vi "Fetch Multi Eval Meas ACLR Detected Allocation Results.vi"(8 "error in (no error)":errorcluster, 10 "Instance (1)":T2=1, 11 "VISA resource name":refnum<visa-resource-name>) -> (0 "error out":errorcluster, 1 "Detected Allocation":T1, 2 "Reliability":i32, 3 "VISA resource name out":refnum<visa-resource-name>)   [LabVIEW 2020, in "Rohde&Schwarz CMWXP NR FR1 Measurement.lvlib"]
doc: "Returns the ACLR detected allocation for the measured slot.\n\nIf the same slot is measured by the individual measurements, all commands yield the same result. If different statistic counts are defined for the modulation, ACLR and spectrum emission mask measurements, different slots can be measured and different results can be returned by the individual commands.\n\nAttribute:\nRSCMWXPNRFR1M_ATTR_FETCH_MULTI_EVAL_MEAS_ACLR_DETECTED_ALLOCATION_RESULTS\n\nRemote-control command:\nFETCh:NRSub:MEAS<i>:MEValuation:ACLR:DALLocation?"
uses:
  <instrlib>/Rohde&Schwarz CMWXP NR FR1 Measurement/Rohde&Schwarz CMWXP NR FR1 Measurement.lvlib
  <instrlib>/Rohde&Schwarz CMWXP NR FR1 Measurement/Private/_Instance.ctl
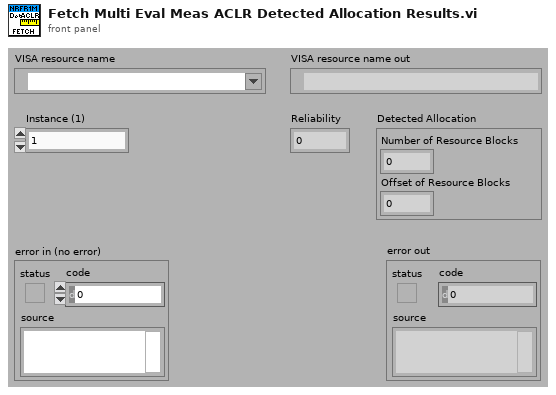
[diagram p1: front panel]
types:
  T1 = cluster{"Number of Resource Blocks":i32, "Offset of Resource Blocks":i32}
  T2 = typedef "Rohde&Schwarz CMWXP NR FR1 Measurement.lvlib/_Instance.ctl" = i32
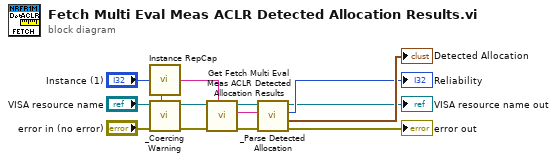
[diagram p0: block diagram]
diagram:
  n1 = call <instrlib>:"Instance RepCap.vi"("Instance In"="Instance (1)") -> ("In Range?"=w11:bool, "RepCap Identifier Out"=w9:string)  [unwired: 1 in]
  n2 = call <instrlib>:"_Coercing Warning.vi"("In Range?"=w11, "error in (no error)"="error in (no error)", "VISA resource name"="VISA resource name") -> ("error out"=w8:errorcluster, "VISA resource name out"=w10:refnum<visa-resource-name>)  [unwired: 7 in]
  n3 = call "Get Fetch Multi Eval Meas ACLR Detected Allocation Results"("Repeated Capabilities"=w9, "error in (no error)"=w8, "instrument handle"=w10) -> ("error out"=w7:errorcluster, "Fetch Multi Eval Meas ACLR Detected Allocation Results"=w5:string, "instrument handle out"=w6:refnum<visa-resource-name>)  [unwired: 6 in]
  n4 = call <instrlib>:"_Parse Detected Allocation.vi"("error in (no error)"=w7, "Input String"=w5, "VISA resource name"=w6) -> ("error out"=→"error out":errorcluster, "Detected Allocation"=→"Detected Allocation":T1, "Reliability"=→"Reliability":i32, "VISA resource name out"=→"VISA resource name out":refnum<visa-resource-name>)  [unwired: 5 in]
